vi "Wheel Pivot.vi"(2 "y in":dbl, 3 "x in":dbl) -> (0 "y out":dbl, 1 "x out":dbl)   [LabVIEW 2018]
panel:
  in  "length/2":dbl=13.75
  in  "width/2":dbl=14.0
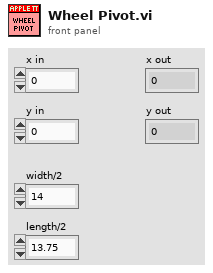
[diagram p1: front panel]
types:
  T1 = cluster{"Yaw":dbl, "Roll":dbl, "Pitch":dbl, "Heading":dbl, "Fused Heading":dbl}
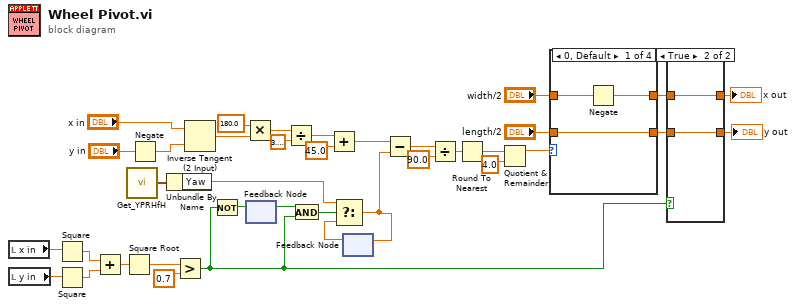
[diagram p0: block diagram]
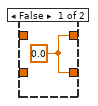
[diagram p2: hidden frame]
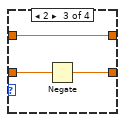
[diagram p4: hidden frame]
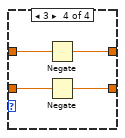
[diagram p5: hidden frame]
diagram:
  n1 = local read "x in"() -> (w20:dbl)
  n2 = local read "y in"() -> (w19:dbl)
  n3 = Square(x=w20) -> (x^2=w18:dbl)
  n4 = Square(x=w19) -> (x^2=w17:dbl)
  n5 = Add(x=w18, y=w17) -> (x+y=w16:dbl)
  n6 = Square Root(x=w16) -> (sqrt(x)=w15:dbl)
  n7 = call <vilib>:"Get_YPRHfH.vi"() -> ("YRPHfH"=w2:T1)  [unwired: 11 in]
  n8 = Negate(x="y in") -> (-x=w30:dbl)
  n9 = Unbundle By Name(w2) -> ("Yaw"=w1:dbl)
  n10 = Greater?(x=w15, y=0.7) -> (0:w7:bool)
  n11 = Inverse Tangent (2 Input)(1:w30, 2:"x in") -> (0:w29:dbl)
  n12 = Not(x=w7) -> (.not. x?=w9:bool)
  n13 = Multiply(x=180.0, y=w29) -> (x*y=w27:dbl)
  n14 = feedback-in #1(w9) -> ()
  n15 = feedback #1() -> (w8:bool)  [unwired: 1 in]
  n16 = Divide(x=w27, y=3.141592653589793) -> (x/y=w23:dbl)
  n17 = And(x=w8, y=w7) -> (x .and. y?=w6:bool)
  n18 = Add(x=w23, y=45.0) -> (x+y=w21:dbl)
  n19 = feedback #2() -> (w5:dbl)  [unwired: 1 in]
  n20 = Select(t=w1, s=w6, f=w5) -> (s? t:f=w3:dbl)
  n21 = feedback-in #2(w3) -> ()
  n22 = Subtract(x=w21, y=w3) -> (x-y=w35:dbl)
  n23 = Divide(x=w35, y=90.0) -> (x/y=w33:dbl)
  n24 = Round To Nearest(number=w33) -> (nearest integer value=w32:dbl)
  n25 = Quotient & Remainder(x=w32, y=4.0) -> (x-y*floor(x/y)=w4:dbl)  [unwired: 1 out]
  n26 = case shown="0, Default" w4 {
    tunnel: "width/2" -> [w40 w42 w43 w49]
    tunnel: "length/2" -> [w38 w41 w45 w47]
    tunnel: [w39 w42 w43 w48] -> w14
    tunnel: [w38 w41 w44 w46] -> w12
    frame 0, Default {
      n27 = Negate(x=w40) -> (-x=w39:dbl)
    }
    frame 1 {
    }
    frame 2 {
      n28 = Negate(x=w45) -> (-x=w44:dbl)
    }
    frame 3 {
      n29 = Negate(x=w49) -> (-x=w48:dbl)
      n30 = Negate(x=w47) -> (-x=w46:dbl)
    }
  }
  n31 = case shown="True" w7 {
    tunnel: w14 -> [_ w52]
    tunnel: [w50 w52] -> w13
    tunnel: w12 -> [_ w51]
    tunnel: [w50 w51] -> w11
    frame False {
      w50 = 0.0 ("y")
    }
    frame True {
    }
  }
  "x out" <- w13
  "y out" <- w11
